vi "Format table.vi"(6 "error in (no error)":errorcluster, 8 "Table Control":string[][](table)=[["aaaa  ", "eeeee", "GGG", ""], ["bbb", "fffffffff", "", ""], ["ccccccc", "", "", ""], ["ddddddddd", "", "", ""], ["", "", "", "I"]], 9 "reference":refnum<vi>) -> (0 "error out":errorcluster)   [LabVIEW 2017]
doc: "this vi is used to resize column widht"
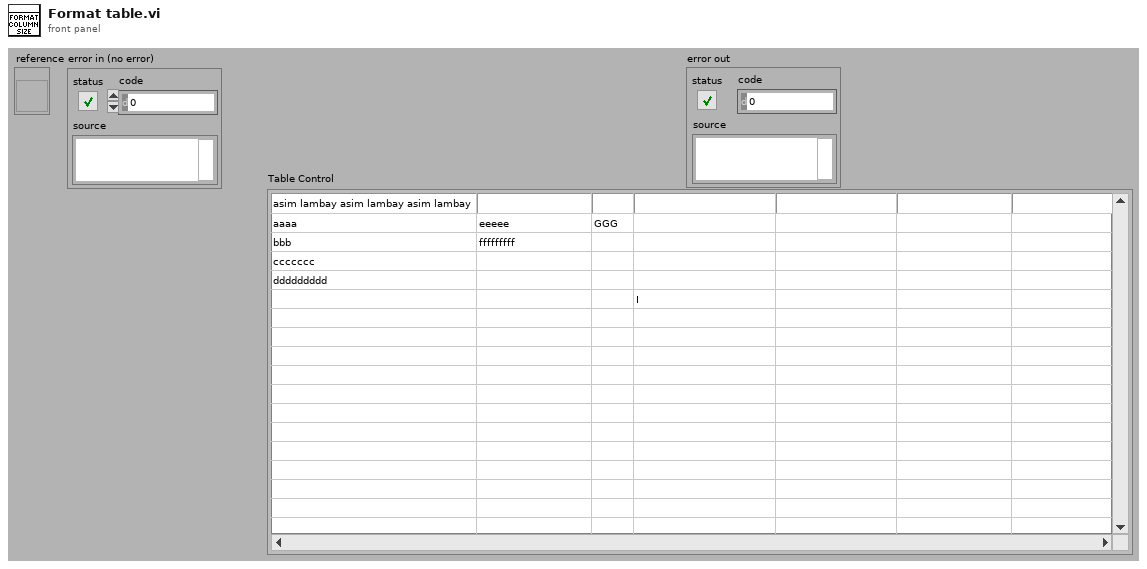
[diagram p1: front panel]
types:
  T1 = cluster{"Font Name:":string, "Size":i16, "Strikeout?":bool, "Italic?":bool, "Underline?":bool, "Outline?":bool, "Shadow?":bool, "Bold?":bool}
  T2 = enum16{"User-specified Font", "Application Font", "System Font", "Dialog Font"}
  T3 = typedef "LVFontTypeDef.ctl" = cluster{"Font Name":string, "Size":u16, "Bold":bool, "Italic":bool, "Underline":bool, "Strikeout":bool, "Color":u32}
  T4 = cluster{"left":i16, "top":i16, "right":i16, "bottom":i16}
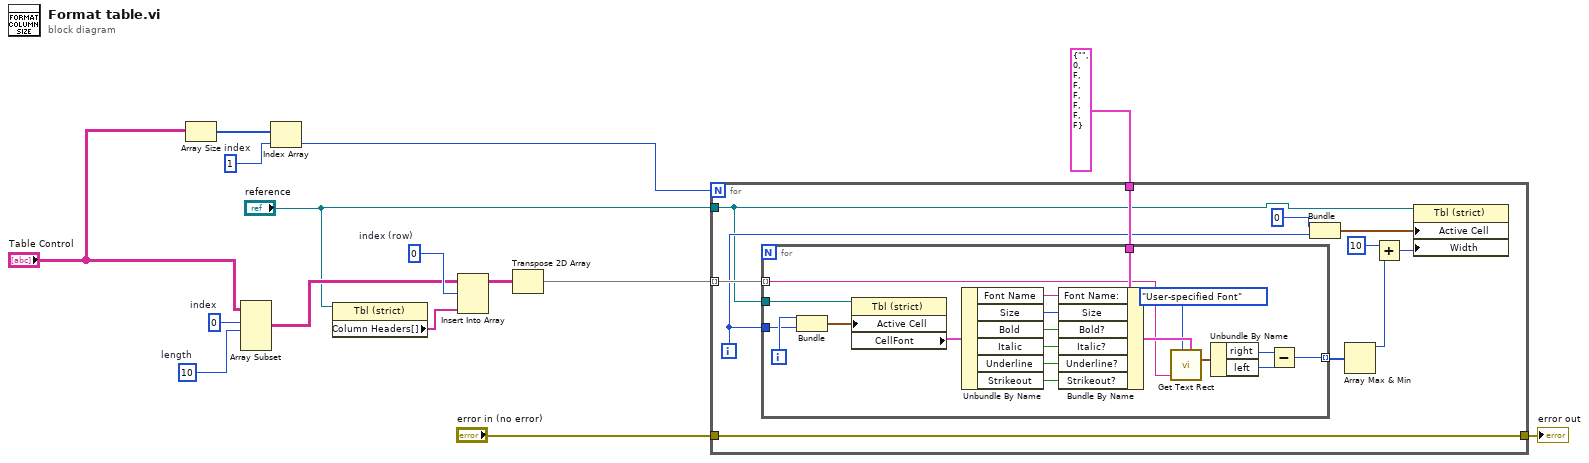
[diagram p0: block diagram]
diagram:
  w5 = 1  # index
  w10 = 10  # length
  w11 = 0  # index
  w14 = 0  # index (row)
  n1 = Array Size(array="Table Control") -> (size(s)=w6:i32[])
  n2 = Array Subset(array="Table Control", index (row)=w11, length (row)=w10) -> (w8:string[][])  [unwired: 2 in]
  n3 = Index Array(array=w6, index=w5) -> (element=w4:i32)
  n4 = property on="Property Node" class="Tbl (strict)"(reference="reference") -> ("Column Headers[]"=w2:string[])  [unwired: 1 in, 2 out]
  n5 = Insert Into Array(array=w8, index (row)=w14, new element=w2) -> (w7:string[][])  [unwired: 1 in]
  n6 = Transpose 2D Array(2D array=w7) -> (transposed array=w9:string[][])
  n7 = for {
    N: w4 -> [_]
    tunnel: w9 -> [w26] mode=indexing
    tunnel: T1 {"Font Name:"="", "Size"=0, "Strikeout?"=FALSE, "Italic?"=FALSE, "Underline?"=FALSE, "Outline?"=FALSE, "Shadow?"=FALSE, "Bold?"=FALSE} ("[user-specified font]") -> [w25]
    tunnel: "reference" -> [w16]
    tunnel: "error in (no error)" -> [w17]
    tunnel: [w17] -> w12
    i -> [w22]
    n8 = for {
      tunnel: w26 -> [w35] mode=indexing
      tunnel: w22 -> [w28]
      tunnel: w25 -> [w43]
      tunnel: [w30] -> w24 mode=indexing
      tunnel: w16 -> [w27]
      i -> [w29]
      n9 = Bundle(w29, w28) -> (w45:cluster{i32, i32})  [unwired: 1 in]
      n10 = property on="Property Node" class="Tbl (strict)"(reference=w27, "Active Cell"=w45) -> ("CellFont"=w42:T3)  [unwired: 1 in, 2 out]
      n11 = Unbundle By Name(w42) -> ("Font Name"=w41:string, "Size"=w40:u16, "Bold"=w39:bool, "Italic"=w38:bool, "Underline"=w37:bool, "Strikeout"=w36:bool)
      n12 = Bundle By Name(cluster=w43, "Font Name:"=w41, "Size"=w40, "Bold?"=w39, "Italic?"=w38, "Underline?"=w37, "Strikeout?"=w36) -> (w44:T1)
      n13 = call <vilib>:"Get Text Rect.vi"("desired font(Application)"=T2."User-specified Font", "text"=w35, "[user-specified font]"=w44) -> ("rect"=w33:T4)  [unwired: 6 in]
      n14 = Unbundle By Name(w33) -> ("right"=w32:i16, "left"=w31:i16)
      n15 = Subtract(x=w32, y=w31) -> (x-y=w30:i16)
    }
    n16 = Bundle(0, w22) -> (w23:cluster{i32, i32})  [unwired: 1 in]
    n17 = Array Max & Min(array=w24) -> (max value=w18:i16)  [unwired: 3 out]
    n18 = Add(x=i16 10, y=w18) -> (x+y=w20:i16)
    n19 = property on="Property Node" class="Tbl (strict)"(reference=w16, "Active Cell"=w23, "Width"=w20) -> ()  [unwired: 1 in, 2 out]
  }
  "error out" <- w12
